vi "Read task config..vi"(11 "settings folder":path) -> (3 "table":string[][](array[string]))   [LabVIEW 2017]
uses:
  <vilib>/Utility/file.llb/Read Delimited Spreadsheet (string).vi
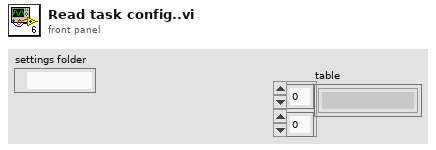
[diagram p1: front panel]
types:
  T1 = enum16{"open", "replace", "create", "open or create", "replace or create", "replace or create with confirmation"}
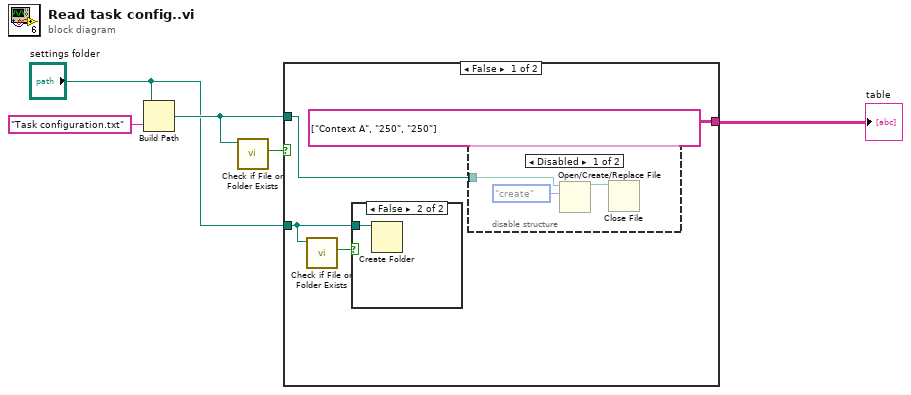
[diagram p0: block diagram]
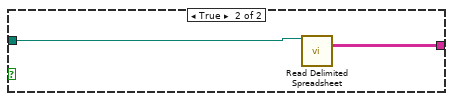
[diagram p4: hidden frame]
diagram:
  n1 = Build Path(base path="settings folder", name or relative path="Task configuration.txt") -> (appended path=w4:path)
  n2 = call <vilib>:"Check if File or Folder Exists.vi"("path"=w4) -> ("file or folder exists?"=w3:bool)  [unwired: 8 in, 2 out]
  n3 = case shown="False" w3 {
    tunnel: w4 -> [w8 w15]
    tunnel: [string[][] [["Context A", "250", "250"]] ("all rows") w14] -> w2
    tunnel: "settings folder" -> [w6 _]
    frame False {
      n4 = call <vilib>:"Check if File or Folder Exists.vi"("path"=w6) -> ("file or folder exists?"=w7:bool)  [unwired: 8 in, 2 out]
      n5 = case shown="False" w7 {
        tunnel: w6 -> [_ w10]
        frame True {
        }
        frame False {
          n6 = Create Folder(path (use dialog)=w10) -> ()  [unwired: 2 in, 3 out]
        }
      }
      n7 = disable-structure shown="Disabled" {
        disable-tunnel: w8 -> [w11 _]
        frame Disabled {
          n8 = Open/Create/Replace File(file path (use dialog)=w11, operation (0:open)=T1."create") -> (refnum out=w12:refnum<file>)  [unwired: 4 in, 2 out]
          n9 = Close File(refnum=w12) -> ()  [unwired: 1 in, 2 out]
        }
        frame Enabled {
        }
      }
    }
    frame True {
      n10 = call-poly <vilib>:"Read Delimited Spreadsheet.vi"("file path (dialog if empty)"=w15) -> ("all rows"=w14:string[][])  [unwired: 9 in, 5 out]
    }
  }
  "table" <- w2
